vi "mp285_GetSta_str2velres.vi"(0 "字符串":string) -> (1 "精度":u16, 2 "速度":dbl)   [LabVIEW 2018]
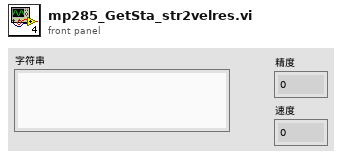
[diagram p1: front panel]
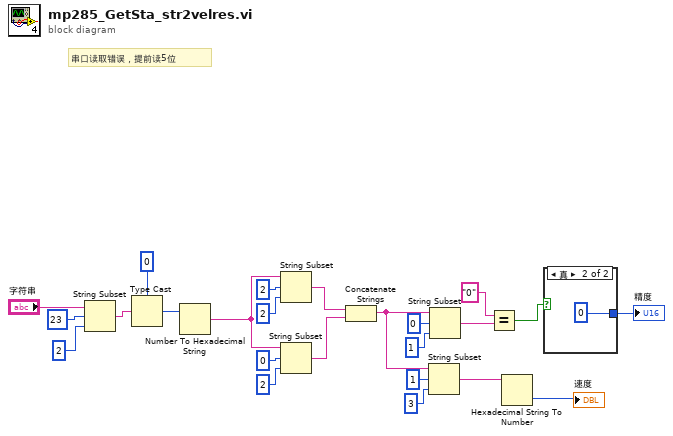
[diagram p0: block diagram]
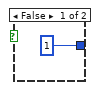
[diagram p2: hidden frame]
diagram:
  # "串口读取错误，提前读5位"
  n1 = String Subset(string="字符串", offset (0)=23 ("偏移量(0)"), length (rest)=2 ("长度（剩余）")) -> (substring=w2:string)
  n2 = Type Cast(type=0, x=w2) -> (*(type *) &x=w4:i32)
  n3 = Number To Hexadecimal String(2:w4) -> (0:w1:string)  [unwired: 1 in]
  n4 = String Subset(string=w1, offset (0)=2 ("偏移量(0)"), length (rest)=2 ("长度（剩余）")) -> (substring=w20:string)
  n5 = String Subset(string=w1, offset (0)=0 ("偏移量(0)"), length (rest)=2 ("长度（剩余）")) -> (substring=w21:string)
  n6 = Concatenate Strings(w20, w21) -> (w13:string)
  n7 = String Subset(string=w13, offset (0)=1 ("偏移量(0)"), length (rest)=3 ("长度（剩余）")) -> (substring=w12:string)
  n8 = String Subset(string=w13, offset (0)=0 ("偏移量(0)"), length (rest)=1 ("长度（剩余）")) -> (substring=w9:string)
  n9 = Equal?(x="0", y=w9) -> (x = y?=w10:bool)
  n10 = Hexadecimal String To Number(string=w12) -> (number=→"速度":u32)  [unwired: 2 in, 1 out]
  n11 = case shown="真" w10 {
    tunnel: [u16 1 ("精度") u16 0 ("精度")] -> w7
    frame False {
    }
    frame True {
    }
  }
  "精度" <- w7
